vi "Write Low Warning Severity.vi"(8 "error in":errorcluster, 10 "low warning severity":T1, 11 "Has Alarm Limits in":refnum<class "Has Alarm Limits.lvclass">) -> (0 "error out":errorcluster, 3 "Has Alarm Limits out":refnum<class "Has Alarm Limits.lvclass">)   [LabVIEW 2020, in "PV Access.lvlib" / "PV Data.lvlib" / "Has Alarm Limits.lvclass"]
uses:
  Has Alarm Limits.lvclass
  Alarm Severity.ctl
  PV Data.lvlib
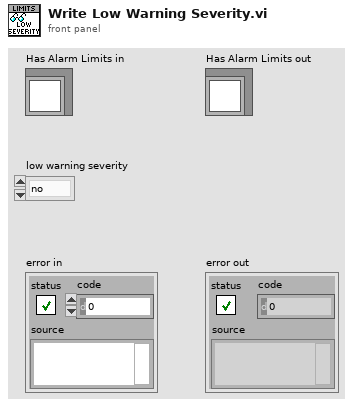
[diagram p1: front panel]
types:
  T1 = typedef "PV Access.lvlib/PV Data.lvlib/Alarm Severity.ctl" = enum32{"no", "minor", "major", "record", "invalid", "undefined"}
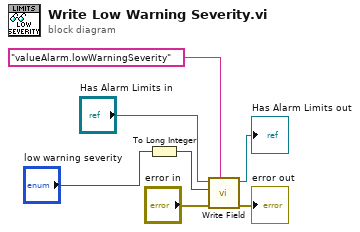
[diagram p0: block diagram]
diagram:
  n1 = To Long Integer(number="low warning severity") -> (32bit integer=w1:i32)
  n2 = call-dynamic "Write Field.vi"("field"="valueAlarm.lowWarningSeverity" ("element name"), "error in (no error)"="error in", "value"=w1, "Base Interface in"="Has Alarm Limits in") -> ("error out"=→"error out":errorcluster, "Base Interface out"=→"Has Alarm Limits out":refnum<class "Has Alarm Limits.lvclass">)  [unwired: 6 in]
